vi "Teleop.vi"(10 "Match Info":T1={"Autonomous Elapsed Seconds"=0.0, "TeleOp Elapsed Seconds"=0.0, "Disabled Elapsed Seconds"=0.0, "Visited Autonomous"=FALSE, "Visited TeleOp"=FALSE, "Visited Disabled"=FALSE, "Autonomous Settings"={"Autonomous Style"=enum."Independent", "VI Refnum"=refnum}}, 11 "Call Context":T2) -> (0 "error out":errorcluster)   [LabVIEW 2019]
doc: "This VI is called for each TeleOp packet received from the DS where the robot is not disabled. It is often used to read from the joysticks and update I/O or to update setpoints for timed control loops. It should complete and return within 20 milliseconds or it may miss DS packets."
uses:
  <vilib>/Rock Robotics/WPI/DriverStation/WPI_DriverStationDerivedRobotMode.ctl
  <vilib>/Rock Robotics/WPI/DriverStation/WPI_DriverStationMatch Info.ctl
  RobotGlobal.vi
  Classes/Joysticks/Joysticks.lvclass
  Classes/Robot/Robot.lvclass
panel:
  in  "error in (no error)":errorcluster
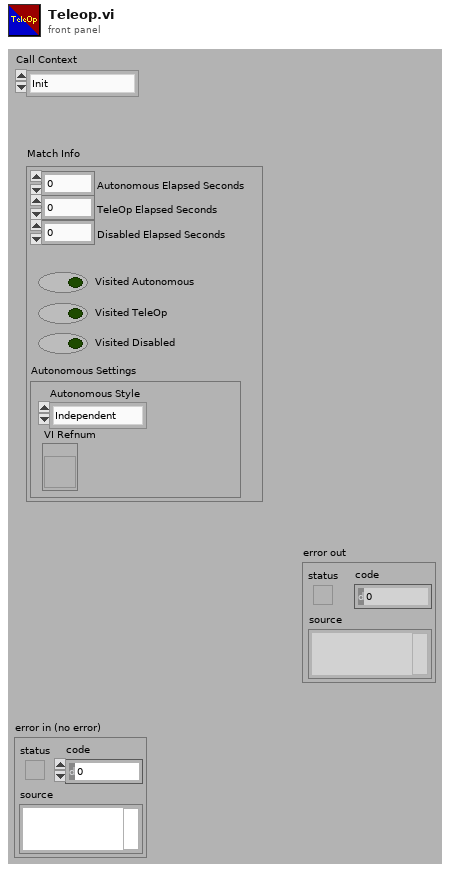
[diagram p1: front panel]
types:
  T1 = typedef "WPI_DriverStationMatch Info.ctl" = cluster{"Autonomous Elapsed Seconds":dbl, "TeleOp Elapsed Seconds":dbl, "Disabled Elapsed Seconds":dbl, "Visited Autonomous":bool, "Visited TeleOp":bool, "Visited Disabled":bool, "Autonomous Settings":cluster{"Autonomous Style":enum16{"Iterative", "Independent"}, "VI Refnum":refnum<vi>}}
  T2 = typedef "WPI_DriverStationDerivedRobotMode.ctl" = enum16{"Init", "Execute", "Stop"}
  T3 = typedef "RobotObjects.ctl" = cluster{"Drive.lvclass":refnum<class "Tank Drive.lvclass">, "Pneumatics.lvclass":refnum<class "Pneumatics.lvclass">, "Vision.lvclass":refnum<class "Vision.lvclass">, "Joysticks.lvclass":refnum<class "Joysticks.lvclass">, "Elevator.lvclass":refnum<class "Elevator.lvclass">, "Hatch.lvclass":refnum<class "Hatch.lvclass">, "Cargo.lvclass":refnum<class "Cargo.lvclass">, "DriveOld.lvclass":refnum<class "Drive.lvclass">, "Robot.lvclass":refnum<class "Robot.lvclass">, "Control Panel.lvclass":refnum<class "Control Panel.lvclass">}
  T4 = typedef "Joysticks.lvlib/Joysticks.lvclass/JoystickData.ctl" = cluster{"X Axis":dbl, "Y Axis":dbl, "Drivetrain Shifter (Hold)":bool, "Beak (Toggle)":bool, "Cargo In (Hold)":bool, "Cargo Out (Hold)":bool, "Switch to hatch(toggle)":bool, "Switch to cargo(toggle)":bool, "Elevator Up (Toggle)":bool, "Elevator Down (Toggle)":bool, "AutoForward (Hold)":bool, "Climb(toggle)":bool, "Disengage Climb(toggle)":bool, "AutoTurn(hold)":bool, "CamMode(Two Driver only)":bool, "AltPipeline":bool}
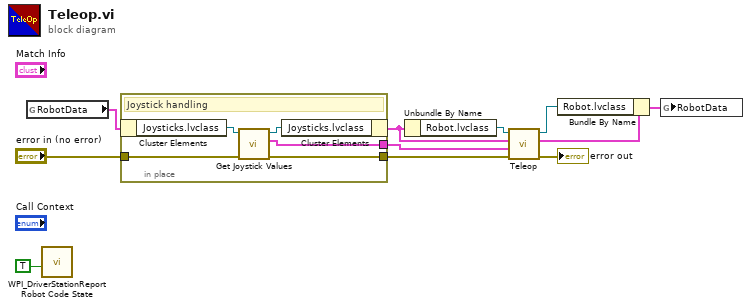
[diagram p0: block diagram]
diagram:
  n1 = global read "RobotGlobal.vi" "RobotData"() -> (w9:T3)
  n2 = call <vilib>:"WPI_DriverStationReport Robot Code State.vi"("TeleOp"=TRUE ("Autonomous")) -> ()  [unwired: 10 in, 1 out]
  n3 = in-place {
    in-place-border: "error in (no error)" -> [w16]
    in-place-border: [w13] -> w7
    in-place-border: [w12] -> w5
    # "Joystick handling"
    n4 = in-place-cluster #1(w9) -> ("Joysticks.lvclass"=w15:refnum<class "Joysticks.lvclass">)
    n5 = call-dynamic "Get Joystick Values.vi"("error in (no error)"=w16, "Joysticks in"=w15) -> ("error out"=w12:errorcluster, "Joystick Data"=w13:T4, "Joysticks out"=w14:refnum<class "Joysticks.lvclass">)  [unwired: 7 in]
    n6 = in-place-cluster #1("Joysticks.lvclass"=w14) -> (w6:T3)
  }
  n7 = Unbundle By Name(w6) -> ("Robot.lvclass"=w8:refnum<class "Robot.lvclass">)
  n8 = call-dynamic "Teleop.vi"("error in (no error)"=w5, "Joystick Data"=w7, "Robot Data In"=w6, "Robot in"=w8) -> ("error out"=→"error out":errorcluster, "Robot Data Out"=w3:T3, "Robot out"=w4:refnum<class "Robot.lvclass">)  [unwired: 5 in]
  n9 = Bundle By Name(cluster=w3, "Robot.lvclass"=w4) -> (w1:T3)
  n10 = global write "RobotGlobal.vi" "RobotData"(w1) -> ()
